vi "Lift Positions.vi"(0 "High":bool, 1 "Middle":bool, 2 "Low":bool, 3 "Bottom":bool, 4 "Top":bool) -> (5 "Clamp Position":dbl)   [LabVIEW 2014]
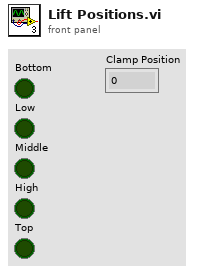
[diagram p1: front panel]
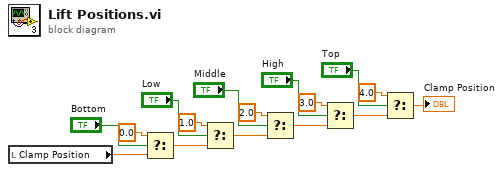
[diagram p0: block diagram]
diagram:
  n1 = local read "Clamp Position"() -> (w6:dbl)
  n2 = Select(t=0.0 ("f"), s="Bottom", f=w6) -> (s? t:f=w8:dbl)
  n3 = Select(t=1.0 ("f"), s="Low", f=w8) -> (s? t:f=w7:dbl)
  n4 = Select(t=2.0, s="Middle", f=w7) -> (s? t:f=w11:dbl)
  n5 = Select(t=3.0, s="High", f=w11) -> (s? t:f=w14:dbl)
  n6 = Select(t=4.0, s="Top", f=w14) -> (s? t:f=→"Clamp Position":dbl)
